vi "Sort Funnels and Paths.vi"(8 "error in (no error)":errorcluster, 11 "Tool Data in":refnum<class "Tool Data.lvclass">) -> (0 "error out":errorcluster, 3 "Tool Data out":refnum<class "Tool Data.lvclass">)   [LabVIEW 2019, in "Tool Data.lvclass"]
uses:
  Tool Data.lvclass
  Parse/ParsePaths/Path.lvclass
  Tool Object/Tool Object.lvclass
  Parse/PathCommands/PathCommands.lvclass
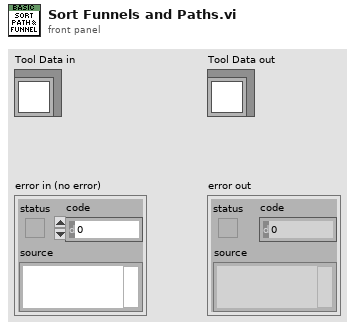
[diagram p1: front panel]
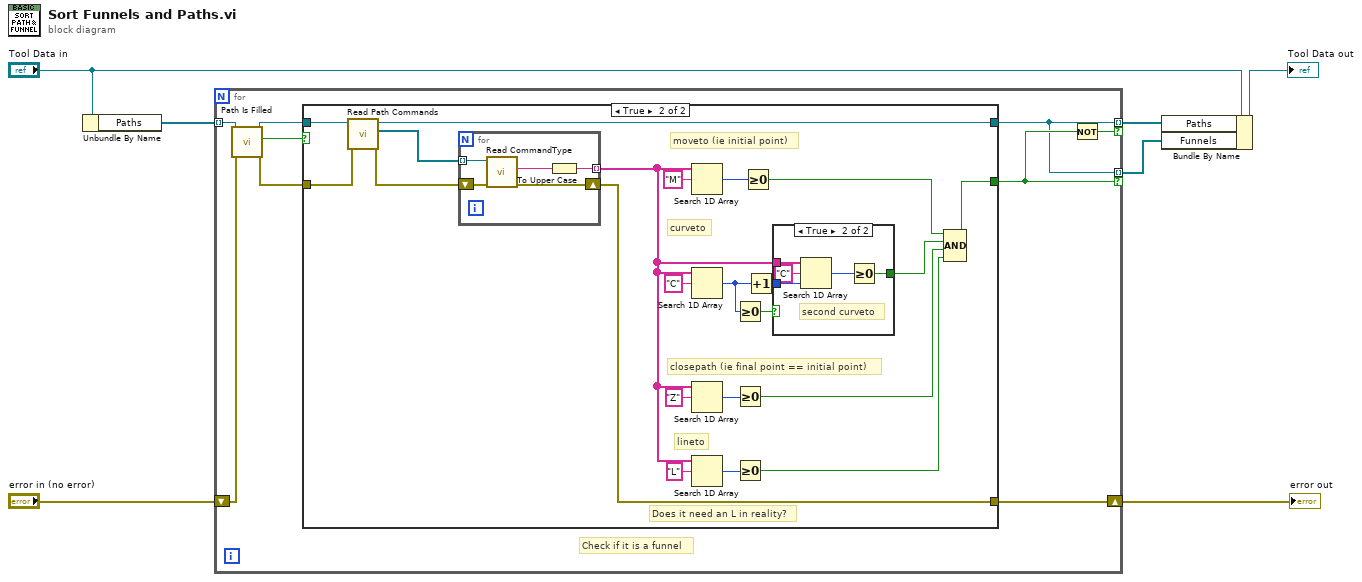
[diagram p0: block diagram]
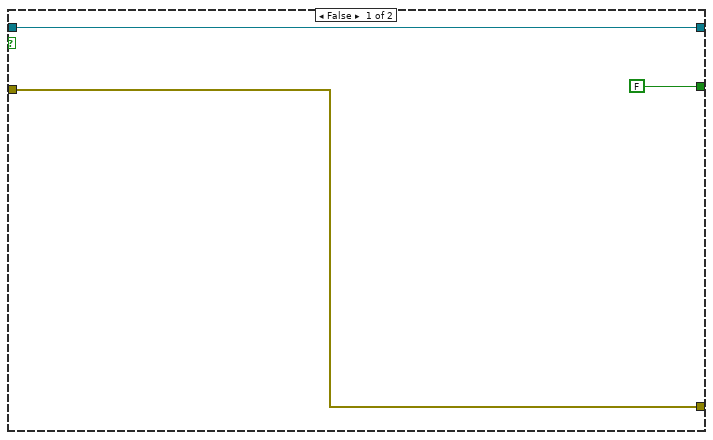
[diagram p2: hidden frame]
diagram:
  n1 = Unbundle By Name("Tool Data in") -> ("Paths"=w7:refnum<class "Path.lvclass">[])
  n2 = for {
    tunnel: w7 -> [w11] mode=indexing
    tunnel: [w14] -> w4 mode=indexing if=w16
    tunnel: [w14] -> w1 mode=indexing if=w15
    shift-right: [w8] -> w5
    shift-left: "error in (no error)" -> [w9]
    # "Check if it is a funnel"
    n3 = call "Path Is Filled.vi"("error in (no error)"=w9, "Path in"=w11) -> ("error out"=w10:errorcluster, "x != y?"=w13:bool, "Path out"=w12:refnum<class "Path.lvclass">)  [unwired: 7 in]
    n4 = case shown="True" w13 {
      tunnel: [FALSE w26] -> w15
      tunnel: w12 -> [w19 w25]
      tunnel: [w19 w24] -> w14
      tunnel: w10 -> [w17 w21]
      tunnel: [w17 w20] -> w8
      frame False {
      }
      frame True {
        # "Does it need an L in reality?"
        # "lineto"
        # "closepath (ie final point == initial point)"
        # "curveto"
        # "moveto (ie initial point)"
        n5 = call "Read Path Commands.vi"("error in (no error)"=w21, "Path in"=w25) -> ("error out"=w22:errorcluster, "Path Commands"=w23:refnum<class "PathCommands.lvclass">[], "Path out"=w24:refnum<class "Path.lvclass">)  [unwired: 7 in]
        n6 = for {
          tunnel: w23 -> [w52] mode=indexing
          tunnel: [w50] -> w27 mode=indexing
          shift-right: [w48] -> w20
          shift-left: w22 -> [w49]
          n7 = call-dynamic "Read CommandType.vi"("error in (no error)"=w49, "PathCommands in"=w52) -> ("error out"=w48:errorcluster, "CommandType"=w51:string)  [unwired: 7 in, 1 out]
          n8 = To Upper Case(1:w51) -> (0:w50:string)
        }
        n9 = Search 1D Array(1D array=w27, element="M") -> (index of element=w39:i32)  [unwired: 1 in]
        n10 = Search 1D Array(1D array=w27, element="C") -> (index of element=w38:i32)  [unwired: 1 in]
        n11 = Search 1D Array(1D array=w27, element="Z") -> (index of element=w35:i32)  [unwired: 1 in]
        n12 = Search 1D Array(1D array=w27, element="L") -> (index of element=w30:i32)  [unwired: 1 in]
        n13 = Greater Or Equal To 0?(x=w38) -> (x >= 0?=w37:bool)
        n14 = Greater Or Equal To 0?(x=w35) -> (x >= 0?=w32:bool)
        n15 = Greater Or Equal To 0?(x=w30) -> (x >= 0?=w28:bool)
        n16 = Greater Or Equal To 0?(x=w39) -> (x >= 0?=w34:bool)
        n17 = Increment(x=w38) -> (x+1=w31:i32)
        n18 = case shown="True" w37 {
          selector: w37 -> [w42 _]
          tunnel: w31 -> [_ w47]
          tunnel: w27 -> [_ w46]
          tunnel: [w42 w44] -> w33
          frame False {
          }
          frame True {
            # "second curveto"
            n19 = Search 1D Array(1D array=w46, element="C", start index (0)=w47) -> (index of element=w45:i32)
            n20 = Greater Or Equal To 0?(x=w45) -> (x >= 0?=w44:bool)
          }
        }
        n21 = Compound Arithmetic op=AND(w34, w33, w32, w28) -> (w26:bool)
      }
    }
    n22 = Not(x=w15) -> (.not. x?=w16:bool)
  }
  "error out" <- w5
  n23 = Bundle By Name(cluster="Tool Data in", "Paths"=w4, "Funnels"=w1) -> (→"Tool Data out":refnum<class "Tool Data.lvclass">)
